vi "Insert Into Subpanel.vi"(7 "View Name":string, 8 "error in (no error)":errorcluster, 9 "Insertion Request Time":timestamp, 10 "VI Refnum":refnum<vi>, 11 "Protected Subpanel":T1) -> (0 "error out":errorcluster, 3 "Protected Subpanel":T1)   [LabVIEW 2015, in "IViewable.lvlib" / "ProtectedSubpanel.lvclass"]
uses:
  ProtectedSubpanel.lvclass
  Protected Subpanel Reference.ctl
  ProtectedSubpanel.lvclass/ProtectedSubpanel.ctl
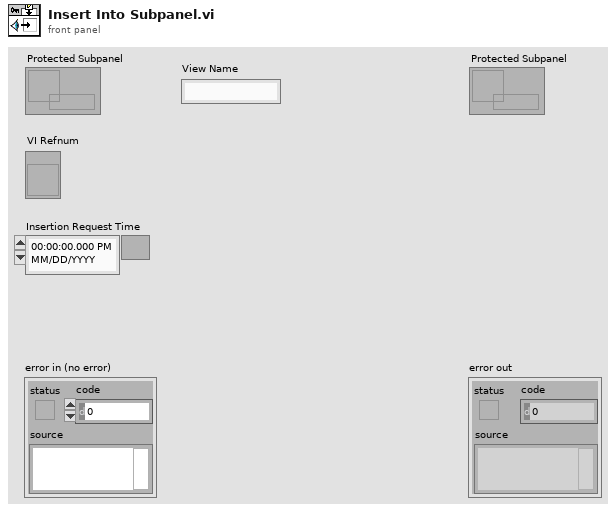
[diagram p1: front panel]
types:
  T1 = typedef "IViewable.lvlib/ProtectedSubpanel.lvclass/Protected Subpanel Reference.ctl" = refnum<data-value>
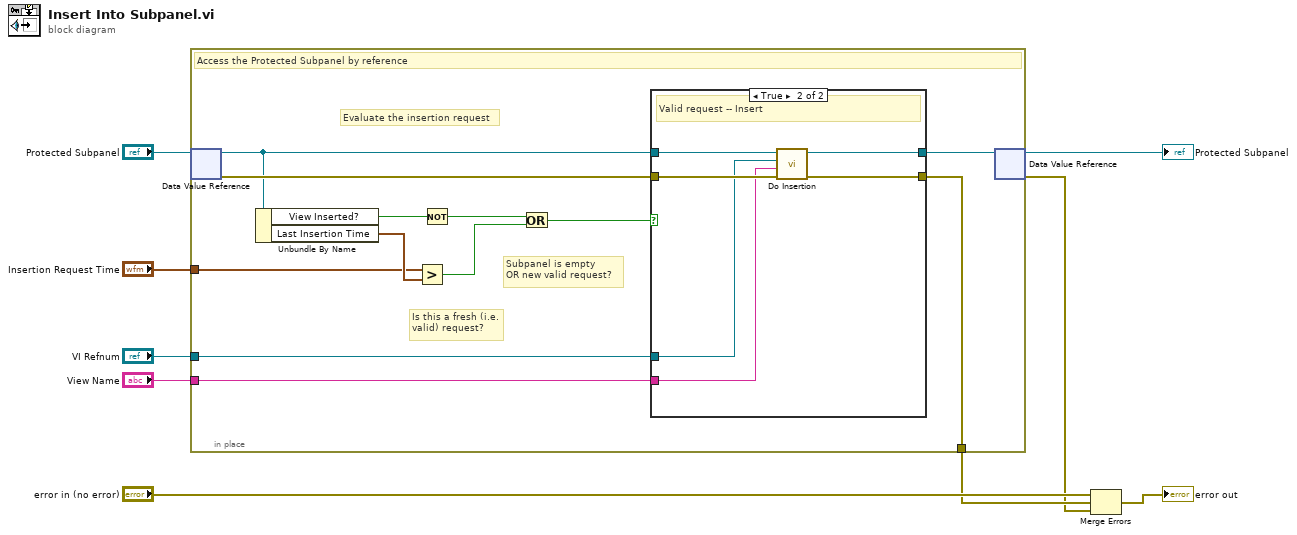
[diagram p0: block diagram]
diagram:
  n1 = in-place {
    in-place-border: "VI Refnum" -> [w20]
    in-place-border: "Insertion Request Time" -> [w12]
    in-place-border: "View Name" -> [w19]
    in-place-border: [w10] -> w2
    # "Evaluate the insertion request"
    # "Subpanel is empty\nOR new valid request?"
    # "Is this a fresh (i.e.\nvalid) request?"
    # "Access the Protected Subpanel by reference"
    n2 = in-place-dvr #1("Protected Subpanel") -> (w11:refnum<class "ProtectedSubpanel.lvclass">, w13:errorcluster)
    n3 = Unbundle By Name(w11) -> ("View Inserted?"=w17:bool, "Last Insertion Time"=w18:timestamp)
    n4 = Greater?(x=w12, y=w18) -> (0:w15:bool)
    n5 = Not(x=w17) -> (.not. x?=w16:bool)
    n6 = Or(x=w16, y=w15) -> (x .or. y?=w14:bool)
    n7 = case shown="True" w14 {
      tunnel: [w23 w29] -> w21
      tunnel: w11 -> [w23 w28]
      tunnel: w13 -> [w22 w27]
      tunnel: [w22 w26] -> w10
      tunnel: w20 -> [_ w25]
      tunnel: w19 -> [_ w24]
      frame False {
        # "Stale request -- No insert"
      }
      frame True {
        # "Valid request -- Insert"
        n8 = call "Do Insertion.vi"("error in (no error)"=w27, "View Name"=w24, "VI Refnum"=w25, "ProtectedSubpanel in"=w28) -> ("error out"=w26:errorcluster, "ProtectedSubpanel out"=w29:refnum<class "ProtectedSubpanel.lvclass">)  [unwired: 6 in]
      }
    }
    n9 = in-place-dvr #1(w21) -> (→"Protected Subpanel":T1, w1:errorcluster)
  }
  n10 = Merge Errors("error in (no error)", w2, w1) -> (→"error out":errorcluster)
